vi "Array_Size_2D.vi"(10 "Array":i8[][](array[numeric])=[[0, 4, 8], [1, 5, 9], [2, 6, 10], [3, 7, 11]]) -> (2 "Size 2D":T1)   [LabVIEW 2018]
uses:
  Controls/Rows_Columns.ctl
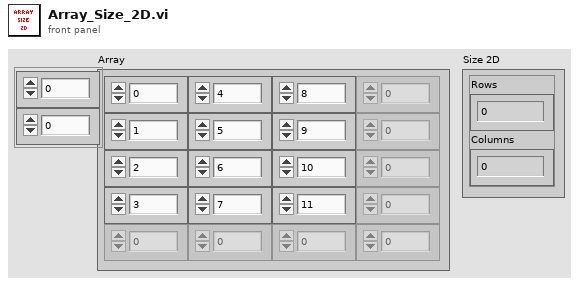
[diagram p1: front panel]
types:
  T1 = typedef "Rows_Columns.ctl" = cluster{"Rows":i32, "Columns":i32}
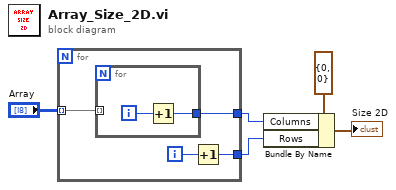
[diagram p0: block diagram]
diagram:
  n1 = for {
    tunnel: "Array" -> [w9] mode=indexing
    tunnel: [w8] -> w5
    tunnel: [w6] -> w4
    i -> [w7]
    n2 = for {
      tunnel: w9 -> [_] mode=indexing
      tunnel: [w10] -> w8
      i -> [w11]
      n3 = Increment(x=w11) -> (x+1=w10:i32)
    }
    n4 = Increment(x=w7) -> (x+1=w6:i32)
  }
  n5 = Bundle By Name(cluster=T1 {"Rows"=0, "Columns"=0} ("Rows & Columns 2"), "Columns"=w5, "Rows"=w4) -> (→"Size 2D":T1)
